vi "LiftQCP.vi"   [LabVIEW 2017]
uses:
  <userlib>/836-Library/System/QCP_V2/QCPSupportCode/QCP_GetDbl.vi
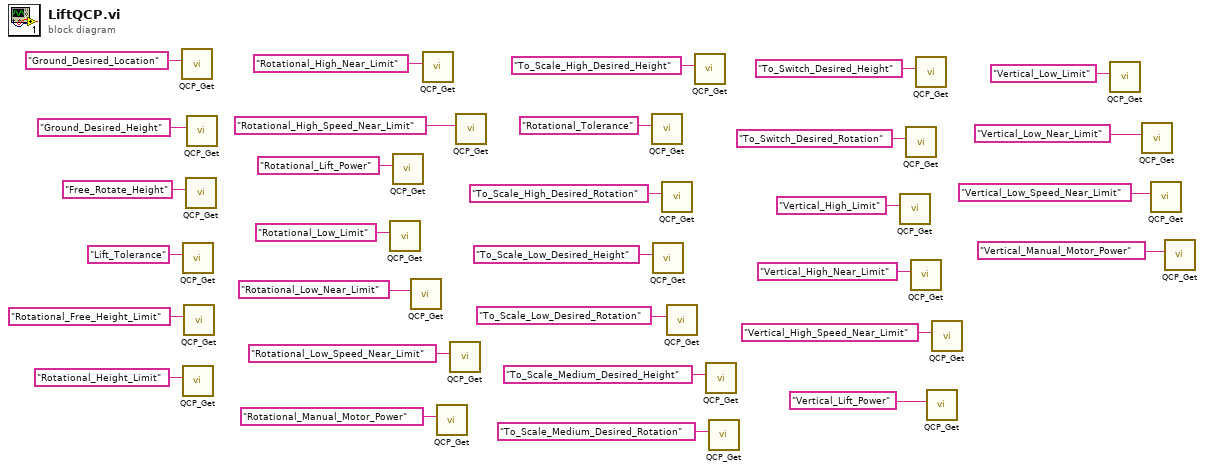
[diagram p0: block diagram]
diagram:
  n1 = call-poly <userlib>:"QCP_Get.vi"("Value Name"="Ground_Desired_Location") -> ()  [unwired: 8 in, 3 out]
  n2 = call-poly <userlib>:"QCP_Get.vi"("Value Name"="Lift_Tolerance") -> ()  [unwired: 8 in, 3 out]
  n3 = call-poly <userlib>:"QCP_Get.vi"("Value Name"="Rotational_Height_Limit") -> ()  [unwired: 8 in, 3 out]
  n4 = call-poly <userlib>:"QCP_Get.vi"("Value Name"="Rotational_Free_Height_Limit") -> ()  [unwired: 8 in, 3 out]
  n5 = call-poly <userlib>:"QCP_Get.vi"("Value Name"="Free_Rotate_Height") -> ()  [unwired: 8 in, 3 out]
  n6 = call-poly <userlib>:"QCP_Get.vi"("Value Name"="Ground_Desired_Height") -> ()  [unwired: 8 in, 3 out]
  n7 = call-poly <userlib>:"QCP_Get.vi"("Value Name"="Rotational_Low_Limit") -> ()  [unwired: 8 in, 3 out]
  n8 = call-poly <userlib>:"QCP_Get.vi"("Value Name"="Rotational_Lift_Power") -> ()  [unwired: 8 in, 3 out]
  n9 = call-poly <userlib>:"QCP_Get.vi"("Value Name"="Rotational_Low_Near_Limit") -> ()  [unwired: 8 in, 3 out]
  n10 = call-poly <userlib>:"QCP_Get.vi"("Value Name"="Rotational_High_Near_Limit") -> ()  [unwired: 8 in, 3 out]
  n11 = call-poly <userlib>:"QCP_Get.vi"("Value Name"="Rotational_Manual_Motor_Power") -> ()  [unwired: 8 in, 3 out]
  n12 = call-poly <userlib>:"QCP_Get.vi"("Value Name"="Rotational_Low_Speed_Near_Limit") -> ()  [unwired: 8 in, 3 out]
  n13 = call-poly <userlib>:"QCP_Get.vi"("Value Name"="Rotational_High_Speed_Near_Limit") -> ()  [unwired: 8 in, 3 out]
  n14 = call-poly <userlib>:"QCP_Get.vi"("Value Name"="Rotational_Tolerance") -> ()  [unwired: 8 in, 3 out]
  n15 = call-poly <userlib>:"QCP_Get.vi"("Value Name"="To_Scale_Low_Desired_Height") -> ()  [unwired: 8 in, 3 out]
  n16 = call-poly <userlib>:"QCP_Get.vi"("Value Name"="To_Scale_High_Desired_Rotation") -> ()  [unwired: 8 in, 3 out]
  n17 = call-poly <userlib>:"QCP_Get.vi"("Value Name"="To_Scale_Low_Desired_Rotation") -> ()  [unwired: 8 in, 3 out]
  n18 = call-poly <userlib>:"QCP_Get.vi"("Value Name"="To_Scale_High_Desired_Height") -> ()  [unwired: 8 in, 3 out]
  n19 = call-poly <userlib>:"QCP_Get.vi"("Value Name"="To_Scale_Medium_Desired_Height") -> ()  [unwired: 8 in, 3 out]
  n20 = call-poly <userlib>:"QCP_Get.vi"("Value Name"="To_Scale_Medium_Desired_Rotation") -> ()  [unwired: 8 in, 3 out]
  n21 = call-poly <userlib>:"QCP_Get.vi"("Value Name"="Vertical_High_Limit") -> ()  [unwired: 8 in, 3 out]
  n22 = call-poly <userlib>:"QCP_Get.vi"("Value Name"="To_Switch_Desired_Rotation") -> ()  [unwired: 8 in, 3 out]
  n23 = call-poly <userlib>:"QCP_Get.vi"("Value Name"="Vertical_High_Near_Limit") -> ()  [unwired: 8 in, 3 out]
  n24 = call-poly <userlib>:"QCP_Get.vi"("Value Name"="To_Switch_Desired_Height") -> ()  [unwired: 8 in, 3 out]
  n25 = call-poly <userlib>:"QCP_Get.vi"("Value Name"="Vertical_Lift_Power") -> ()  [unwired: 8 in, 3 out]
  n26 = call-poly <userlib>:"QCP_Get.vi"("Value Name"="Vertical_High_Speed_Near_Limit") -> ()  [unwired: 8 in, 3 out]
  n27 = call-poly <userlib>:"QCP_Get.vi"("Value Name"="Vertical_Low_Limit") -> ()  [unwired: 8 in, 3 out]
  n28 = call-poly <userlib>:"QCP_Get.vi"("Value Name"="Vertical_Low_Near_Limit") -> ()  [unwired: 8 in, 3 out]
  n29 = call-poly <userlib>:"QCP_Get.vi"("Value Name"="Vertical_Low_Speed_Near_Limit") -> ()  [unwired: 8 in, 3 out]
  n30 = call-poly <userlib>:"QCP_Get.vi"("Value Name"="Vertical_Manual_Motor_Power") -> ()  [unwired: 8 in, 3 out]
